vi "dvp Vi Set Noise Reduct2d State.vi"(10 "NoiseReduct2dState":i32, 11 "handle":u32) -> (3 "function return":u32(ring))   [LabVIEW 2018, in "LabViewDVPCamera.lvlib"]
doc: "LabviewDvp2Api dvpStatus dvpViSetNoiseReduct2dState(dvpHandle handle, BOOL NoiseReduct2dState);"
uses:
  LabViewDVPCamera.lvlib
  LabViewDVPCamera/LabViewDVPCamera.dll
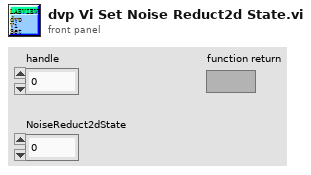
[diagram p1: front panel]
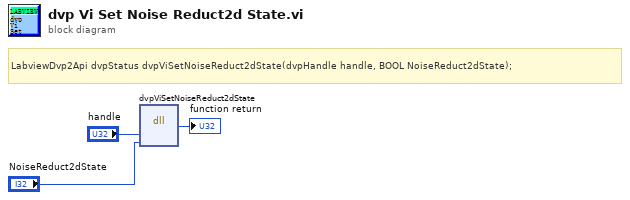
[diagram p0: block diagram]
diagram:
  # "LabviewDvp2Api dvpStatus dvpViSetNoiseReduct2dState(dvpHandle handle, BOOL NoiseReduct2dState);"
  n1 = dll-call lib="C:/Program Files (x86)/DVP2 Labview cn 64/Sample/LabViewDVPCamera/LabViewDVPCamera.*" fn="dvpViSetNoiseReduct2dState"("handle"="handle", "NoiseReduct2dState"="NoiseReduct2dState") -> (→"function return":u32)  [unwired: 5 in, 2 out]
